vi "显示列表行数.vi"(10 "显示行数":i32, 11 "接收数据列表":string[][](array[string])) -> (3 "输出簇":T1)   [LabVIEW 2015, in "下位机模拟.lvlib" / "下位机模拟.lvclass"]
uses:
  <vilib>/Utility/miscctls.llb/LVRowAndColumnUnsignedTypeDef.ctl
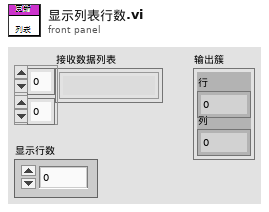
[diagram p1: front panel]
types:
  T1 = typedef "LVRowAndColumnUnsignedTypeDef.ctl" = cluster{"Row":u32, "Column":u32}
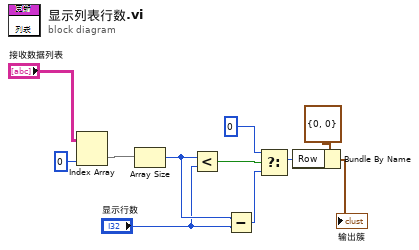
[diagram p0: block diagram]
diagram:
  n1 = Index Array(array="接收数据列表", index (col)=0 ("禁用的索引 (列)")) -> (element=w6:string[])  [unwired: 1 in]
  n2 = Array Size(array=w6) -> (size(s)=w4:i32)
  n3 = Less?(x=w4, y="显示行数") -> (x < y?=w7:bool)
  n4 = Subtract(x=w4, y="显示行数") -> (x-y=w2:i32)
  n5 = Select(t=0 ("大小"), s=w7, f=w2) -> (s? t:f=w10:i32)
  n6 = Bundle By Name(cluster=T1 {"Row"=0, "Column"=0} ("左上可见单元格"), "Row"=w10) -> (→"输出簇":T1)
